vi "SendUserEventMessage_Cluster.vi"(8 "error in":errorcluster, 10 "message":T1, 11 "message ref in":refnum<class "CLM_LocalMessage_UserEvent.lvclass">) -> (0 "error out":errorcluster, 3 "message ref out":refnum<class "CLM_LocalMessage_UserEvent.lvclass">)   [LabVIEW 2013, in "CLM_LocalMessage_UserEvent.lvclass"]
uses:
  CLM_LocalMessage_UserEvent.lvclass
  LocalMessage/Message.ctl
  <vilib>/event_ctls.llb/usereventprio.ctl
  CLM_LocalMessage_UserEvent.lvclass/CLM_LocalMessage_UserEvent.ctl
  LocalMessage/CLM_LocalMessage.lvclass
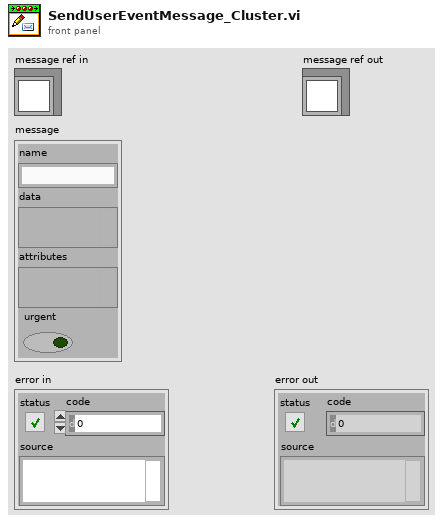
[diagram p1: front panel]
types:
  T1 = typedef "CLM_LocalMessage.lvclass/Message.ctl" = cluster{"name":string, "data":variant, "attributes":variant, "urgent":bool}
  T2 = typedef "usereventprio.ctl" = enum32{"high priority", "normal priority"}
  T3 = typedef "CLM_LocalMessage_UserEvent.lvclass/MessageUserEvent.ctl" = refnum<user-event>
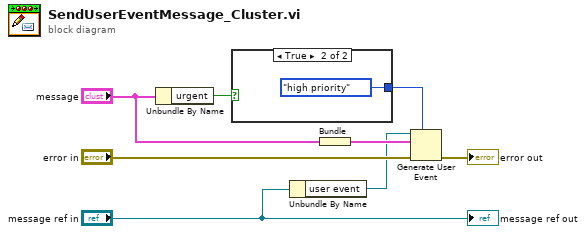
[diagram p0: block diagram]
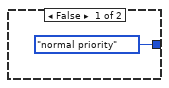
[diagram p2: hidden frame]
diagram:
  n1 = Unbundle By Name("message") -> ("urgent"=w8:bool)
  n2 = case shown="True" w8 {
    tunnel: [usereventprio."normal priority" ("priority (normal)") usereventprio."high priority" ("priority (normal)")] -> w7
    frame False {
    }
    frame True {
    }
  }
  n3 = Unbundle By Name("message ref in") -> ("user event"=w1:T3)
  n4 = Bundle("message"="message") -> (w3:cluster{"message":T1})  [unwired: 1 in]
  n5 = Generate User Event(priority (normal)=w7, user event=w1, event data cluster=w3, error in="error in") -> (error out=→"error out":errorcluster)  [unwired: 1 out]
  "message ref out" <- "message ref in"
